vi "KISSIA__MIDE_FLUJOS.vi"(6 "error in (no error)":errorcluster, 7 "Index":i8) -> (0 "error out":errorcluster, 2 "resulting string 1":string="Mide Bronkhorst 1, mide Alicats 1,  y pausa 1.0s", 3 "Cancelled?":bool)   [LabVIEW 2017]
doc: "Use this template to create a dialog box. This template polls the state of the buttons on the front panel and does not use events. Use the Dialog Using Events template (not available in Base package) to create a dialog box with event handling."
panel:
  in  "Mide Bronkhorst":bool=TRUE
  in  "Pausa (s)":dbl=1.0
  in  "Mide Alicats":bool=TRUE
  in  "Cancel":bool
  in  "OK":bool
  # "MEDIR FLUJOS"
  # "Noviembre 2022 V1.0  a-sslcdms"
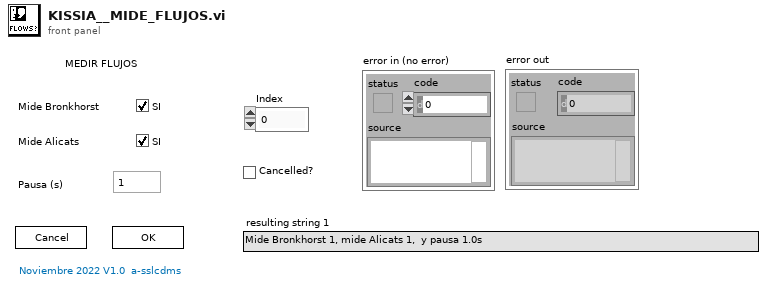
[diagram p1: front panel]
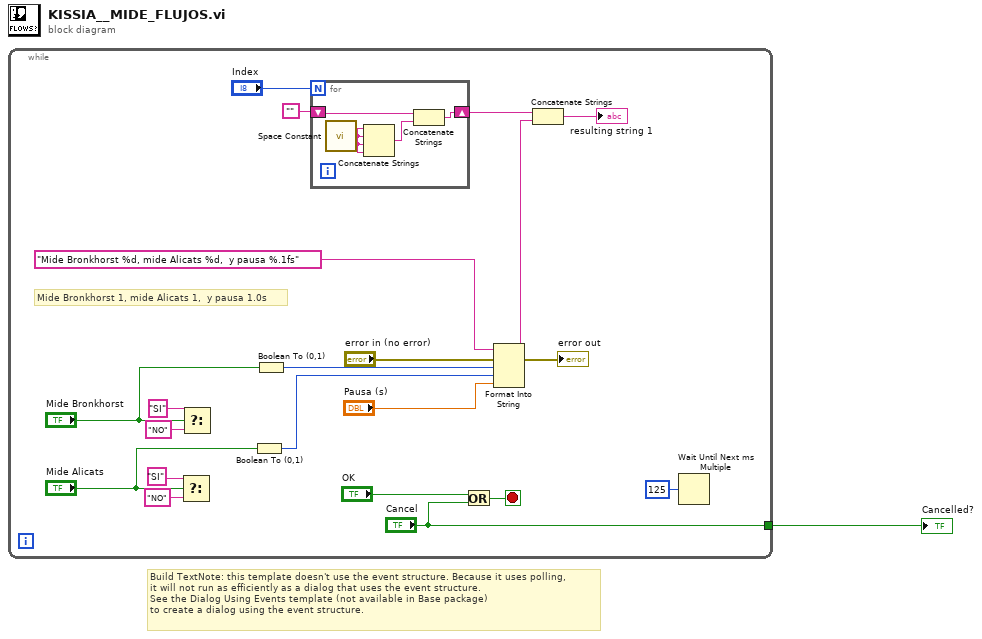
[diagram p0: block diagram]
diagram:
  # "Build TextNote: this template doesn't use the event structure. Because it uses polling, \nit will not run as efficiently as a dialog that uses the event structure.\nSee the Dialog Using Events template (not available in Base package) \nto create a dialog using the event structure."
  n1 = while {
    tunnel: ["Cancel"] -> w1
    stop <- w21 stop-if-true
    # "Mide Bronkhorst 1, mide Alicats 1,  y pausa 1.0s"
    n2 = Select(t="SI", s="Mide Alicats", f="NO") -> ()  [unwired: 1 out]
    n3 = Select(t="SI", s="Mide Bronkhorst", f="NO") -> ()  [unwired: 1 out]
    n4 = Boolean To (0,1)(Boolean="Mide Alicats") -> (0, 1=w5:i16)
    n5 = Boolean To (0,1)(Boolean="Mide Bronkhorst") -> (0, 1=w4:i16)
    n6 = for {
      N: "Index" -> [_]
      shift-right: [w25] -> w13
      shift-left: "" -> [w24]
      n7 = call <vilib>:"Space Constant.vi"() -> ("String"=w23:string)
      n8 = Concatenate Strings(w23, w23, w23, w23) -> (w26:string)
      n9 = Concatenate Strings(w24, w26) -> (w25:string)
    }
    n10 = Or(x="OK", y="Cancel") -> (x .or. y?=w21:bool)
    n11 = Format Into String(format string="Mide Bronkhorst %d, mide Alicats %d,  y pausa %.1fs", error in="error in (no error)", w4, w5, "Pausa (s)") -> (resulting string=w9:string, error out=→"error out":errorcluster)  [unwired: 1 in]
    n12 = Concatenate Strings(w13, w9) -> (→"resulting string 1":string)
    n13 = Wait Until Next ms Multiple(millisecond multiple=u32 125) -> ()  [unwired: 1 out]
  }
  "Cancelled?" <- w1
